vi "Get All Filters.vi"(8 "error in (no error)":errorcluster, 11 "Bus Monitor in":refnum<class "Bus Monitor.lvclass">) -> (0 "error out":errorcluster, 1 "Filters":refnum<class "Filter.lvclass">[](array[class]), 2 "Filter IDs":string[](array[string]), 3 "Bus Monitor out":refnum<class "Bus Monitor.lvclass">)   [LabVIEW 2020, in "BCI-1553 API.lvlib" / "Bus Monitor.lvclass"]
doc: "Retrieves all the filters and filter IDs from this Bus Monitor."
uses:
  Bus Monitor.lvclass
  Filters/Filter/Filter.lvclass
  Bus Monitor.lvclass/Bus Monitor.ctl
  Dependencies/Registry/Registry.lvclass/Registry.ctl
  Dependencies/Registry/Registry.lvclass
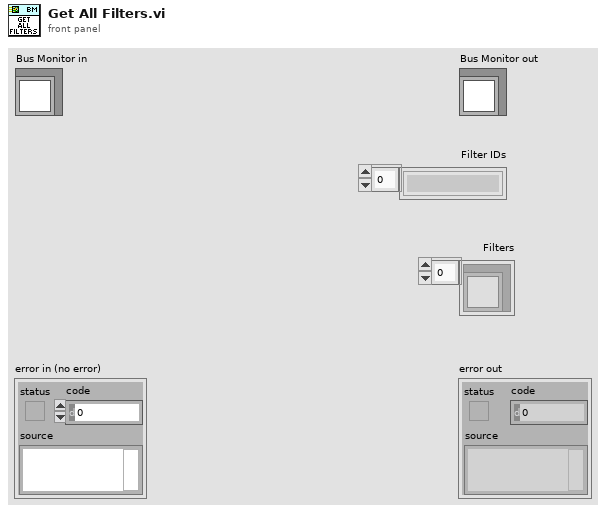
[diagram p1: front panel]
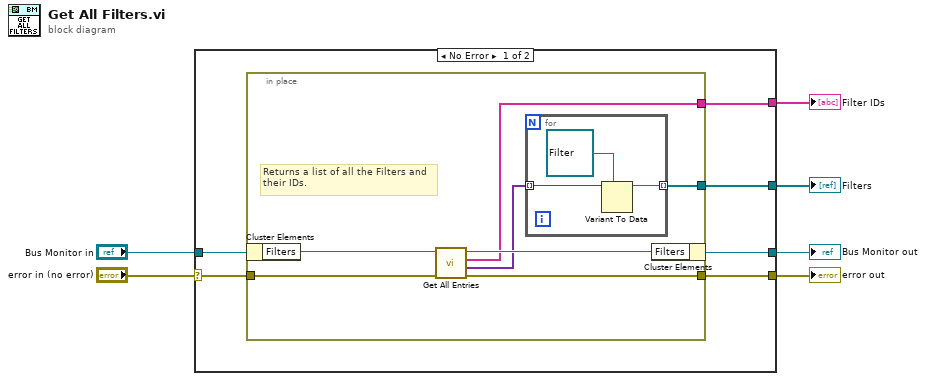
[diagram p0: block diagram]
diagram:
  n1 = case shown="No Error" "error in (no error)" {
    selector: "error in (no error)" -> [w9 w23]
    tunnel: [w10 w23] -> w4
    tunnel: [w11 w22] -> w3
    tunnel: "Bus Monitor in" -> [w12 w22]
    tunnel: [w8 _] -> w2
    tunnel: [w7 _] -> w1
    frame No Error {
      n2 = in-place {
        in-place-border: [w16] -> w10
        in-place-border: w9 -> [w17]
        in-place-border: [w15] -> w7
        in-place-border: [w13] -> w8
        # "Returns a list of all the Filters and\ntheir IDs."
        n3 = in-place-cluster #1(w12) -> ("Filters"=w18:refnum<class "Registry.lvclass">)
        n4 = call "Get All Entries.vi"("error in (no error)"=w17, "Registry in"=w18) -> ("error out"=w16:errorcluster, "Values"=w14:variant[], "Keys"=w15:string[])  [unwired: 7 in]
        n5 = for {
          tunnel: w14 -> [w21] mode=indexing
          tunnel: [w20] -> w13 mode=indexing
          n6 = Variant To Data(type=refnum<class "Filter.lvclass"> refnum ("SLSC 1553 API.lvlib:Filter.lvclass"), Variant=w21) -> (data=w20:refnum<class "Filter.lvclass">)  [unwired: 1 in, 1 out]
        }
        n7 = in-place-cluster #1("Filters"=w18) -> (w11:refnum<class "Bus Monitor.lvclass">)
      }
    }
    frame Error {
    }
  }
  "error out" <- w4
  "Bus Monitor out" <- w3
  "Filters" <- w2
  "Filter IDs" <- w1
